vi "colors.vi"() -> ()   [LabVIEW 2021]
panel:
  in  "Colors":T1={"primary color"=3289650, "secondary color"=6776679, "accent color"=15213, "background color"=16185078, "accent s color"=15213}
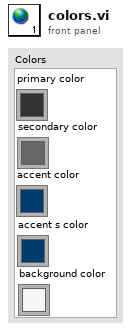
[diagram p1: front panel]
types:
  T1 = cluster{"primary color":u32, "secondary color":u32, "accent color":u32, "background color":u32, "accent s color":u32}
diagram:
